vi "USD Coins.vi"(8 "error in (no error)":errorcluster, 10 "Coins":cluster{"1":bool, "2":bool, "5":bool}, 11 "USD Actor in":refnum<class "USD Actor.lvclass">) -> (0 "error out":errorcluster, 3 "USD Actor out":refnum<class "USD Actor.lvclass">)   [LabVIEW 2020, in "USD Actor.lvlib" / "USD Actor.lvclass"]
uses:
  USD Actor.lvclass
  C:/Program Files (x86)/National Instruments/LabVIEW 2020/vi.lib/ActorFramework/Actor/Actor.lvclass
  <vilib>/ActorFramework/Actor/Actor.lvclass/Actor.ctl
  USD Actor.lvclass/USD Actor.ctl
  UI Actor Messages/Credit Update Msg/Credit Update Msg.lvclass/Credit Update Msg.ctl
  <vilib>/ActorFramework/Message Enqueuer/Message Enqueuer.lvclass/Message Enqueuer.ctl
  <vilib>/ActorFramework/Message Enqueuer/Enqueue.vi
  UI Actor Messages/Credit Update Msg/Credit Update Msg.lvclass
  C:/Program Files (x86)/National Instruments/LabVIEW 2020/vi.lib/ActorFramework/Message/Message.lvclass
  <vilib>/ActorFramework/Message Priority Queue/Priority Enqueue.vi
  <vilib>/ActorFramework/Actor/Actor.lvclass
panel:
  # "USD"
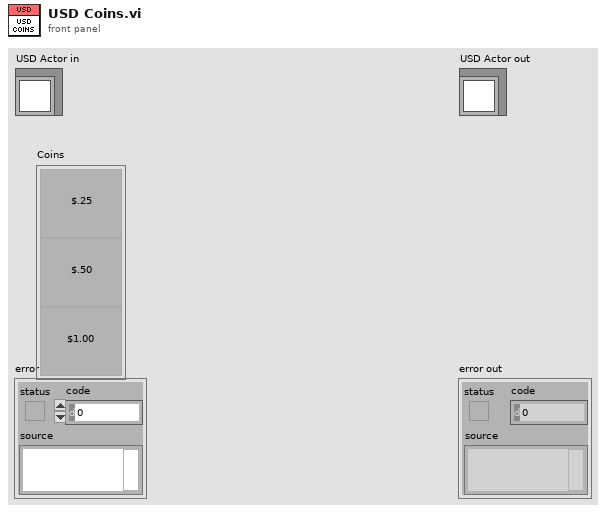
[diagram p1: front panel]
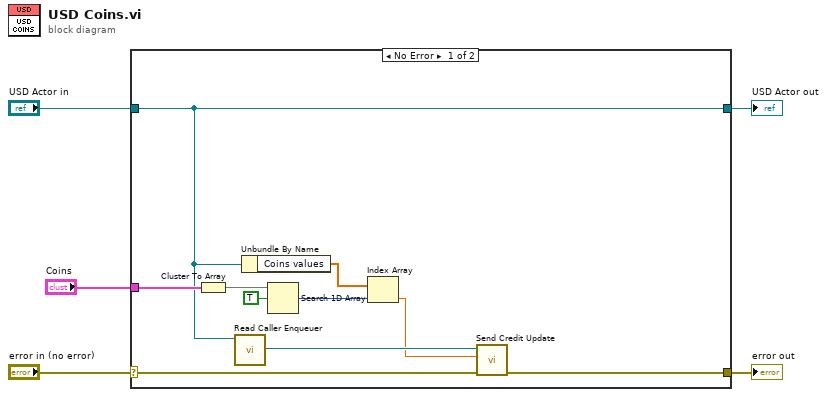
[diagram p0: block diagram]
diagram:
  n1 = case shown="No Error" "error in (no error)" {
    selector: "error in (no error)" -> [w7 w17]
    tunnel: [w6 w17] -> w4
    tunnel: [w8 w16] -> w2
    tunnel: "USD Actor in" -> [w8 w16]
    tunnel: "Coins" -> [w9 _]
    frame No Error {
      n2 = Cluster To Array(cluster=w9) -> (array=w15:bool[])
      n3 = call <vilib>:"Read Caller Enqueuer.vi"("Actor"=w8) -> ("Caller Enqueuer"=w11:refnum<class "Message Enqueuer.lvclass">)  [unwired: 10 in]
      n4 = Unbundle By Name(w8) -> ("Coins values"=w13:dbl[])
      n5 = Search 1D Array(1D array=w15, element=TRUE) -> (index of element=w12:i32)  [unwired: 1 in]
      n6 = Index Array(array=w13, index=w12) -> (element=w10:dbl)
      n7 = call "Send Credit Update.vi"("error in (no error)"=w7, "Credit"=w10, "Message Enqueuer"=w11) -> ("error out"=w6:errorcluster)  [unwired: 7 in, 1 out]
    }
    frame Error {
    }
  }
  "error out" <- w4
  "USD Actor out" <- w2
